vi "Send MoveAfterReference.vi"(7 "Message Priority (Normal)":T1=enum."Normal", 8 "error in (no error)":errorcluster, 9 "Position":dbl, 10 "AxisNumber":u8, 11 "Message Enqueuer":refnum<class "Message Enqueuer.lvclass">) -> (0 "error out":errorcluster, 3 "Message Enqueuer out":refnum<class "Message Enqueuer.lvclass">)   [LabVIEW 2015, in "CS++Motor.lvlib" / "MoveAfterReference Msg.lvclass"]
doc: "Sends the <B>CS++Motor.lvlib:MoveAfterReference Msg.lvclass</B> message.\n\n<B>CS++Motor.lvlib:CS++Motor.lvclass:MoveAfterReference.vi</B> Description:\n\nStarts a movement to the reference switch of this axis. Once the motor reaches the reference switch it should slowly move down from the switch, resets the internal step counter and moves to the desired absolute position.\n\nThis function is a combination of <b>Move.vi</b> and <b>ReferenceMove.vi</b>."
uses:
  MoveAfterReference Msg.lvclass
  <vilib>/ActorFramework/Message Enqueuer/Message Enqueuer.lvclass
  <vilib>/ActorFramework/Message Enqueuer/Message Priority.ctl
  MoveAfterReference Msg.lvclass/MoveAfterReference Msg.ctl
  <vilib>/ActorFramework/Message Enqueuer/Message Enqueuer.lvclass/Message Enqueuer.ctl
  <vilib>/ActorFramework/Message Priority Queue/Priority Enqueue.vi
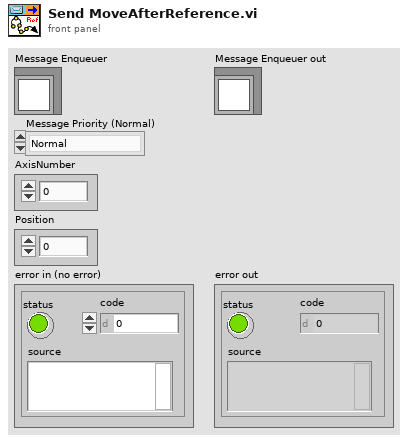
[diagram p1: front panel]
types:
  T1 = typedef "Actor Framework.lvlib/Message Enqueuer.lvclass/Message Priority.ctl" = enum16{"Low", "Normal", "High"}
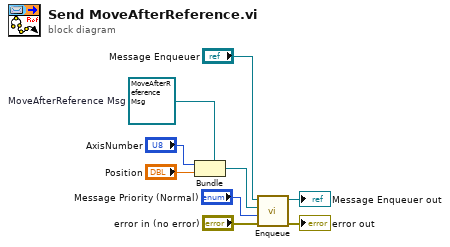
[diagram p0: block diagram]
diagram:
  w3 = refnum<class "MoveAfterReference Msg.lvclass"> refnum  # MoveAfterReference Msg
  n1 = Bundle(cluster=w3, "AxisNumber", "Position") -> (w6:refnum<class "MoveAfterReference Msg.lvclass">)
  n2 = call <vilib>:"Enqueue.vi"("error in (no error)"="error in (no error)", "Message Priority (Normal)"="Message Priority (Normal)", "Message"=w6, "Message Enqueuer in"="Message Enqueuer") -> ("error out"=→"error out":errorcluster, "Message Enqueuer out"=→"Message Enqueuer out":refnum<class "Message Enqueuer.lvclass">)  [unwired: 6 in]
